vi "Get Object Size.vi"   [LabVIEW 2016, in "Data Sharing Framework.Runtime.lvlib"]
uses:
  Data Sharing Framework.Runtime.lvlib
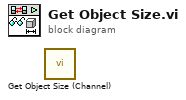
[diagram p0: block diagram]
diagram:
  n1 = call "Get Object Size (Channel).vi"() -> ()  [unwired: 10 in, 2 out]
